vi "MonocromatorControl.vi"(2 "error in (no error)":errorcluster, 3 "Wavelength:":i16, 4 "ComPort:":refnum<visa-resource-name>) -> (0 "Error Out":errorcluster, 1 "return count":u32)   [LabVIEW 2014]
uses:
  <vilib>/Instr/_visa.llb/VISA Configure Serial Port (Instr).vi
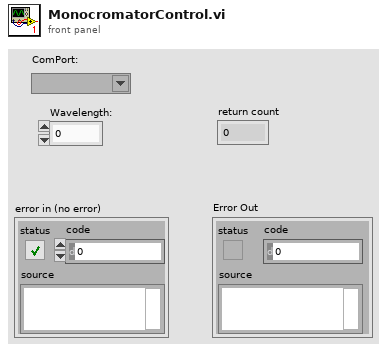
[diagram p1: front panel]
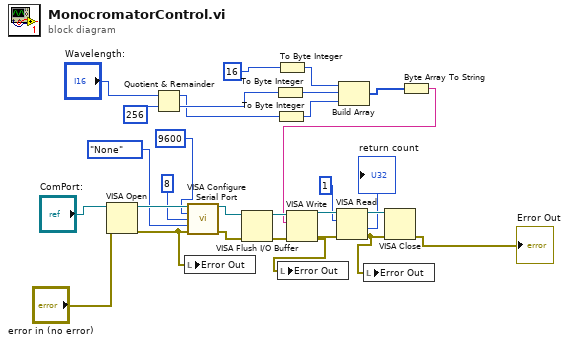
[diagram p0: block diagram]
diagram:
  n1 = VISA Open(error in (no error)="error in (no error)", VISA resource name="ComPort:") -> (VISA resource name=w26:refnum<visa-resource-name>, error out=w23:errorcluster)  [unwired: 3 in]
  n2 = Quotient & Remainder(x="Wavelength:", y=i16 256) -> (x-y*floor(x/y)=w8:i16, floor(x/y)=w9:i16)
  n3 = local write "Error Out"(w23) -> ()
  n4 = call-poly "VISA Configure Serial Port"("VISA resource name"=w26, "baud rate (9600)"=u32 9600, "data bits (8)"=u16 8, "parity (0:none)"=enum16{"None", "Odd", "Even", "Mark", "Space"}."None", "error in (no error)"=w23) -> ("VISA resource name out"=w25:refnum<visa-resource-name>, "error out"=w24:errorcluster)  [unwired: 9 in]
  n5 = VISA Flush I/O Buffer(VISA resource name=w25, error in (no error)=w24) -> (VISA resource name out=w27:refnum<visa-resource-name>, error out=w28:errorcluster)  [unwired: 1 in]
  n6 = To Byte Integer(number=w9) -> (8bit integer=w15:i8)
  n7 = To Byte Integer(number=w8) -> (8bit integer=w16:i8)
  n8 = To Byte Integer(number=u32 16) -> (8bit integer=w14:i8)
  n9 = Build Array(w14, w15, w16) -> (w13:i8[])
  n10 = Byte Array To String(unsigned byte array=w13) -> (string=w12:string)
  n11 = VISA Write(VISA resource name=w27, write buffer=w12, error in (no error)=w28) -> (VISA resource name out=w5:refnum<visa-resource-name>, error out=w6:errorcluster)  [unwired: 1 out]
  n12 = local write "Error Out"(w6) -> ()
  n13 = VISA Read(VISA resource name=w5, byte count=u32 1, error in (no error)=w6) -> (VISA resource name out=w4:refnum<visa-resource-name>, return count=→"return count":u32, error out=w3:errorcluster)  [unwired: 1 out]
  n14 = local write "Error Out"(w3) -> ()
  n15 = VISA Close(VISA resource name=w4, error in (no error)=w3) -> (error out=→"Error Out":errorcluster)
